vi "Com_Panel_Panel Run Time Mode.vi"(8 "error in":errorcluster, 11 "VI Refnum In":refnum<vi>) -> (0 "error out":errorcluster, 3 "VI RefnumOut":refnum<vi>)   [LabVIEW 2016]
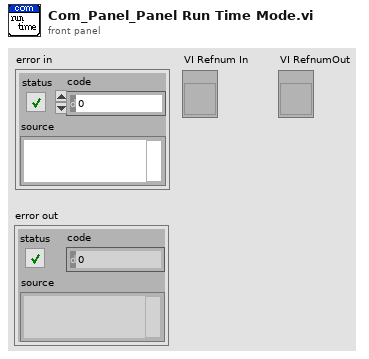
[diagram p1: front panel]
types:
  T1 = enum32{"Invalid", "Standard", "Closed", "Hidden", "Minimized", "Maximized"}
  T2 = enum16{"Always On", "Always Off", "Off While Running"}
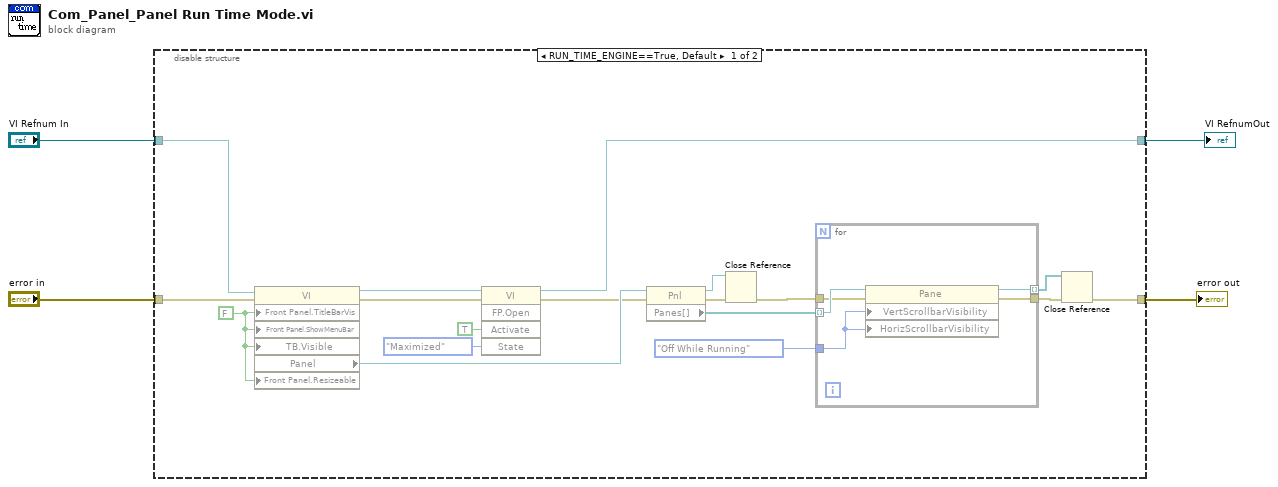
[diagram p0: block diagram]
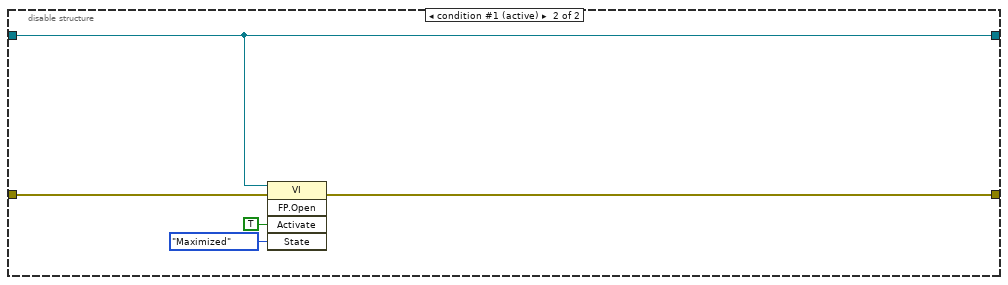
[diagram p2: hidden frame]
diagram:
  n1 = disable-structure shown="RUN_TIME_ENGINE==True, Default" {
    disable-tunnel: "error in" -> [w22 w30]
    disable-tunnel: "VI Refnum In" -> [w21 w28]
    disable-tunnel: [w12 w29] -> w2
    disable-tunnel: [w7 w28] -> w1
    frame condition #0 {
      w11 = FALSE ("Front Panel Window:Title Bar Visible")
      n2 = property class="VI"(reference=w21, error in=w22, "Front Panel.TitleBarVis"=w11, "Front Panel.ShowMenuBar"=w11, "TB.Visible"=w11, "Front Panel.Resizeable"=w11) -> (reference out=w9:refnum<vi>, error out=w10:errorcluster, "Panel"=w20:refnum<vi>)
      n3 = invoke class="VI" method="FP.Open"(reference=w9, error in=w10, "Activate"=TRUE ("Activate?"), "State"=T1."Maximized") -> (reference out=w7:refnum<vi>, error out=w8:errorcluster)  [unwired: 1 in, 3 out]
      n4 = property class="Pnl"(reference=w20, error in=w8) -> (reference out=w17:refnum<vi>, error out=w18:errorcluster, "Panes[]"=w19:refnum<vi>[])
      n5 = Close Reference(reference=w17, error in (no error)=w18) -> (error out=w16:errorcluster)
      n6 = for {
        tunnel: w19 -> [w27] mode=indexing
        tunnel: w16 -> [w26]
        tunnel: T2."Off While Running" ("Horizontal Scrollbar Visibility") -> [w25]
        tunnel: [w24] -> w14
        tunnel: [w23] -> w13 mode=indexing
        n7 = property class="Pane"(reference=w27, error in=w26, "VertScrollbarVisibility"=w25, "HorizScrollbarVisibility"=w25) -> (reference out=w23:refnum<vi>, error out=w24:errorcluster)
      }
      n8 = Close Reference(reference=w13, error in (no error)=w14) -> (error out=w12:errorcluster)
    }
    frame condition #1 (active) {
      n9 = invoke class="VI" method="FP.Open"(reference=w28, error in=w30, "Activate"=TRUE ("Activate?"), "State"=T1."Maximized") -> (error out=w29:errorcluster)  [unwired: 1 in, 4 out]
    }
  }
  "error out" <- w2
  "VI RefnumOut" <- w1
